vi "例8.4 利用DAQmx函数连续模入.vi"() -> ()   [LabVIEW 2017]
uses:
  <vilib>/DAQmx/read.llb/DAQmx Read (Analog 2D DBL NChan NSamp).vi
  <vilib>/DAQmx/create/channels.llb/DAQmx Create Channel (AI-Voltage-Basic).vi
  <vilib>/DAQmx/configure/timing.llb/DAQmx Timing (Sample Clock).vi
  <vilib>/DAQmx/miscellaneous.llb/DAQmx Fill In Error Info.vi
panel:
  in  "samples per channel":i32=1000 caption="每通道采样"
  in  "停止":bool
  out "波形图表":dbl[][](graph)
  out "波形图":dbl[][](graph)
  in  "number of samples per channel":i32=-1 caption="每通道采样数"
  in  "sample mode":i32(ring)=10123 caption="采样模式" items=["有限采样"=10178, "连续采样"=10123, "硬件定时单点"=12522]
  in  "rate":dbl=1000.0 caption="采样率" format="%0.2f"
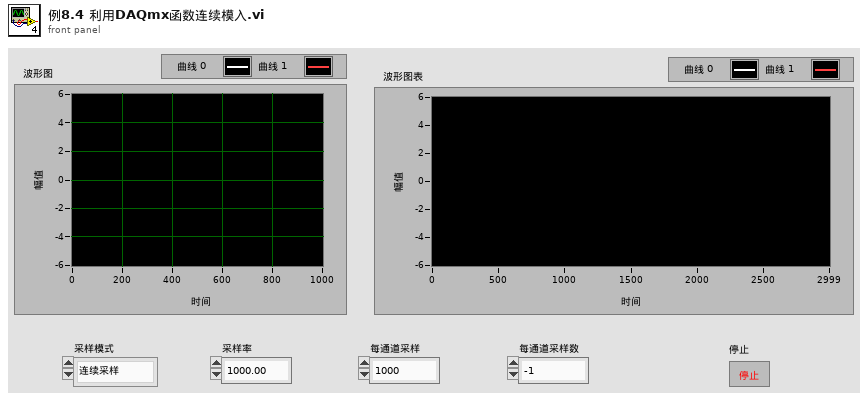
[diagram p1: front panel]
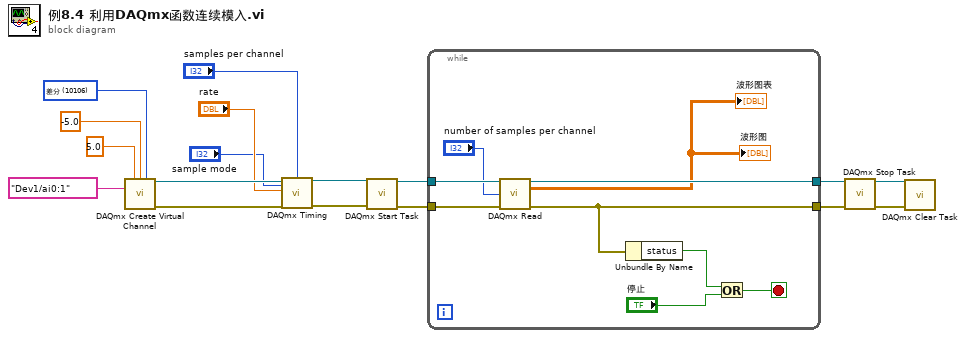
[diagram p0: block diagram]
diagram:
  w7 = 10106 items=["默认"=-1, "RSE"=10083, "NRSE"=10078, "差分"=10106, "伪差分"=12529] ("input terminal configuration")
  n1 = call-poly <vilib>:"DAQmx Create Virtual Channel.vi"("maximum value"=5.0, "minimum value"=-5.0, "input terminal configuration"=w7, "physical channels"=tag "Dev1/ai0:1") -> ("task out"=w17:refnum<k21>, "error out"=w12:errorcluster)  [unwired: 10 in]
  n2 = call-poly <vilib>:"DAQmx Timing.vi"("task/channels in"=w17, "sample mode"="sample mode", "samples per channel"="samples per channel", "rate"="rate", "error in"=w12) -> ("task out"=w16:refnum<k21>, "error out"=w11:errorcluster)  [unwired: 9 in]
  n3 = call <vilib>:"DAQmx Start Task.vi"("task/channels in"=w16, "error in"=w11) -> ("task out"=w15:refnum<k21>, "error out"=w10:errorcluster)  [unwired: 12 in]
  n4 = while {
    tunnel: w15 -> [w26]
    tunnel: [w25] -> w14
    tunnel: w10 -> [w24]
    tunnel: [w21] -> w9
    stop <- w18 stop-if-true
    n5 = call-poly <vilib>:"DAQmx Read.vi"("task/channels in"=w26, "number of samples per channel"="number of samples per channel", "error in"=w24) -> ("task out"=w25:refnum<k21>, "data"=→"波形图表" →"波形图":dbl[][], "error out"=w21:errorcluster)  [unwired: 10 in]
    n6 = Unbundle By Name(w21) -> ("status"=w20:bool)
    n7 = Or(x=w20, y="停止") -> (x .or. y?=w18:bool)
  }
  n8 = call <vilib>:"DAQmx Stop Task.vi"("task/channels in"=w14, "error in"=w9) -> ("task out"=w13:refnum<k21>, "error out"=w8:errorcluster)  [unwired: 12 in]
  n9 = call <vilib>:"DAQmx Clear Task.vi"("task in"=w13, "error in"=w8) -> ()  [unwired: 13 in, 1 out]
